vi "Delete Definition.vi"(7 "Type":string, 8 "error in (no error)":errorcluster, 10 "Name":string, 11 "InsightCM Console Wrapper in":refnum<class "InsightCM Console Wrapper.lvclass">) -> (0 "error out":errorcluster, 3 "InsightCM Console Wrapper out":refnum<class "InsightCM Console Wrapper.lvclass">)   [LabVIEW 2020, in "InsightCM Console Wrapper.lvclass"]
doc: "Excludes a specific definition. You need to enter both type and name of the definition.\n\nConsole commands -> deletedefinition -t [type] -n [name]"
uses:
  InsightCM Console Wrapper.lvclass
  C:/Users/fflores/Documents/GitHub Projects/LabVIEW-CLI-Wrapper/Console Wrapper/Console Wrapper.lvclass
  Console Wrapper/Console Wrapper.lvclass/Console Wrapper.ctl
  Console Wrapper/Write Command Options.vi
  Console Wrapper/Write Command.vi
  Console Wrapper/Console Wrapper.lvclass
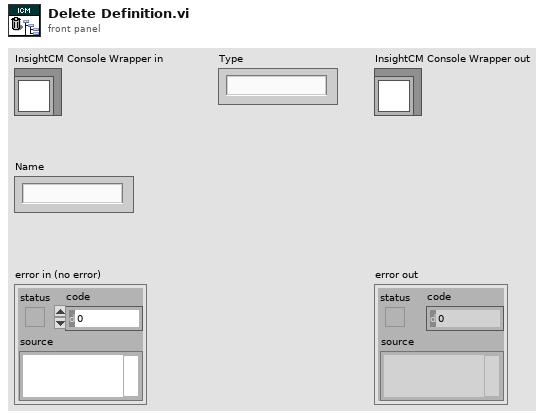
[diagram p1: front panel]
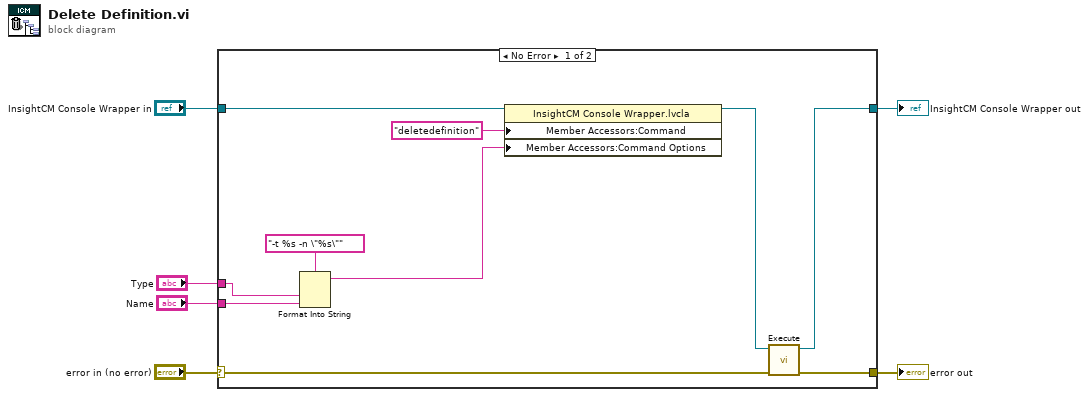
[diagram p0: block diagram]
diagram:
  n1 = case shown="No Error" "error in (no error)" {
    selector: "error in (no error)" -> [w16 w18]
    tunnel: [w15 w18] -> w5
    tunnel: [w13 w17] -> w3
    tunnel: "InsightCM Console Wrapper in" -> [w14 w17]
    tunnel: "Name" -> [w8 _]
    tunnel: "Type" -> [w9 _]
    frame No Error {
      n2 = Format Into String(format string="-t %s -n \"%s\"", w9, w8) -> (resulting string=w7:string)  [unwired: 2 in, 1 out]
      n3 = property class="InsightCM Console Wrapper.lvcla"(reference=w14, "Member Accessors:Command"="deletedefinition" ("Command"), "Member Accessors:Command Options"=w7) -> (reference out=w12:refnum<class "InsightCM Console Wrapper.lvclass">)  [unwired: 1 in, 1 out]
      n4 = call "Execute.vi"("error in (no error)"=w16, "Console Wrapper in"=w12) -> ("error out"=w15:errorcluster, "Console Wrapper out"=w13:refnum<class "InsightCM Console Wrapper.lvclass">)  [unwired: 7 in, 1 out]
    }
    frame Error {
    }
  }
  "error out" <- w5
  "InsightCM Console Wrapper out" <- w3
